vi "TCP_open.vi"(9 "timeout ms":i32=10000 caption="超时毫秒", 11 "Port":u16=2011 caption="端口") -> (0 "error IO":errorcluster, 1 "remote port":u16 caption="远程端口", 2 "remote address":string caption="远程地址", 3 "connection ID":refnum<k5>)   [LabVIEW 2013]
panel:
  # "通信接中～～～"
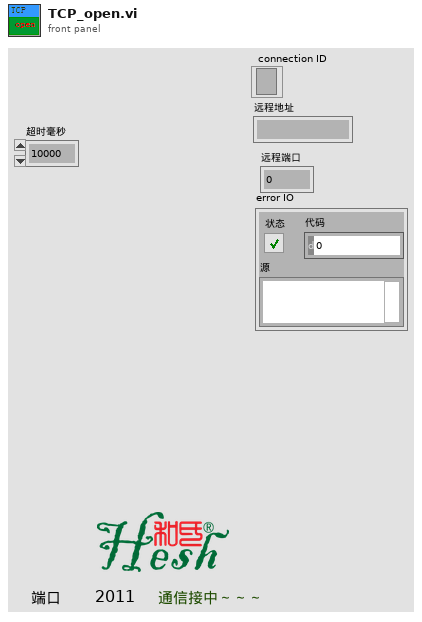
[diagram p1: front panel]
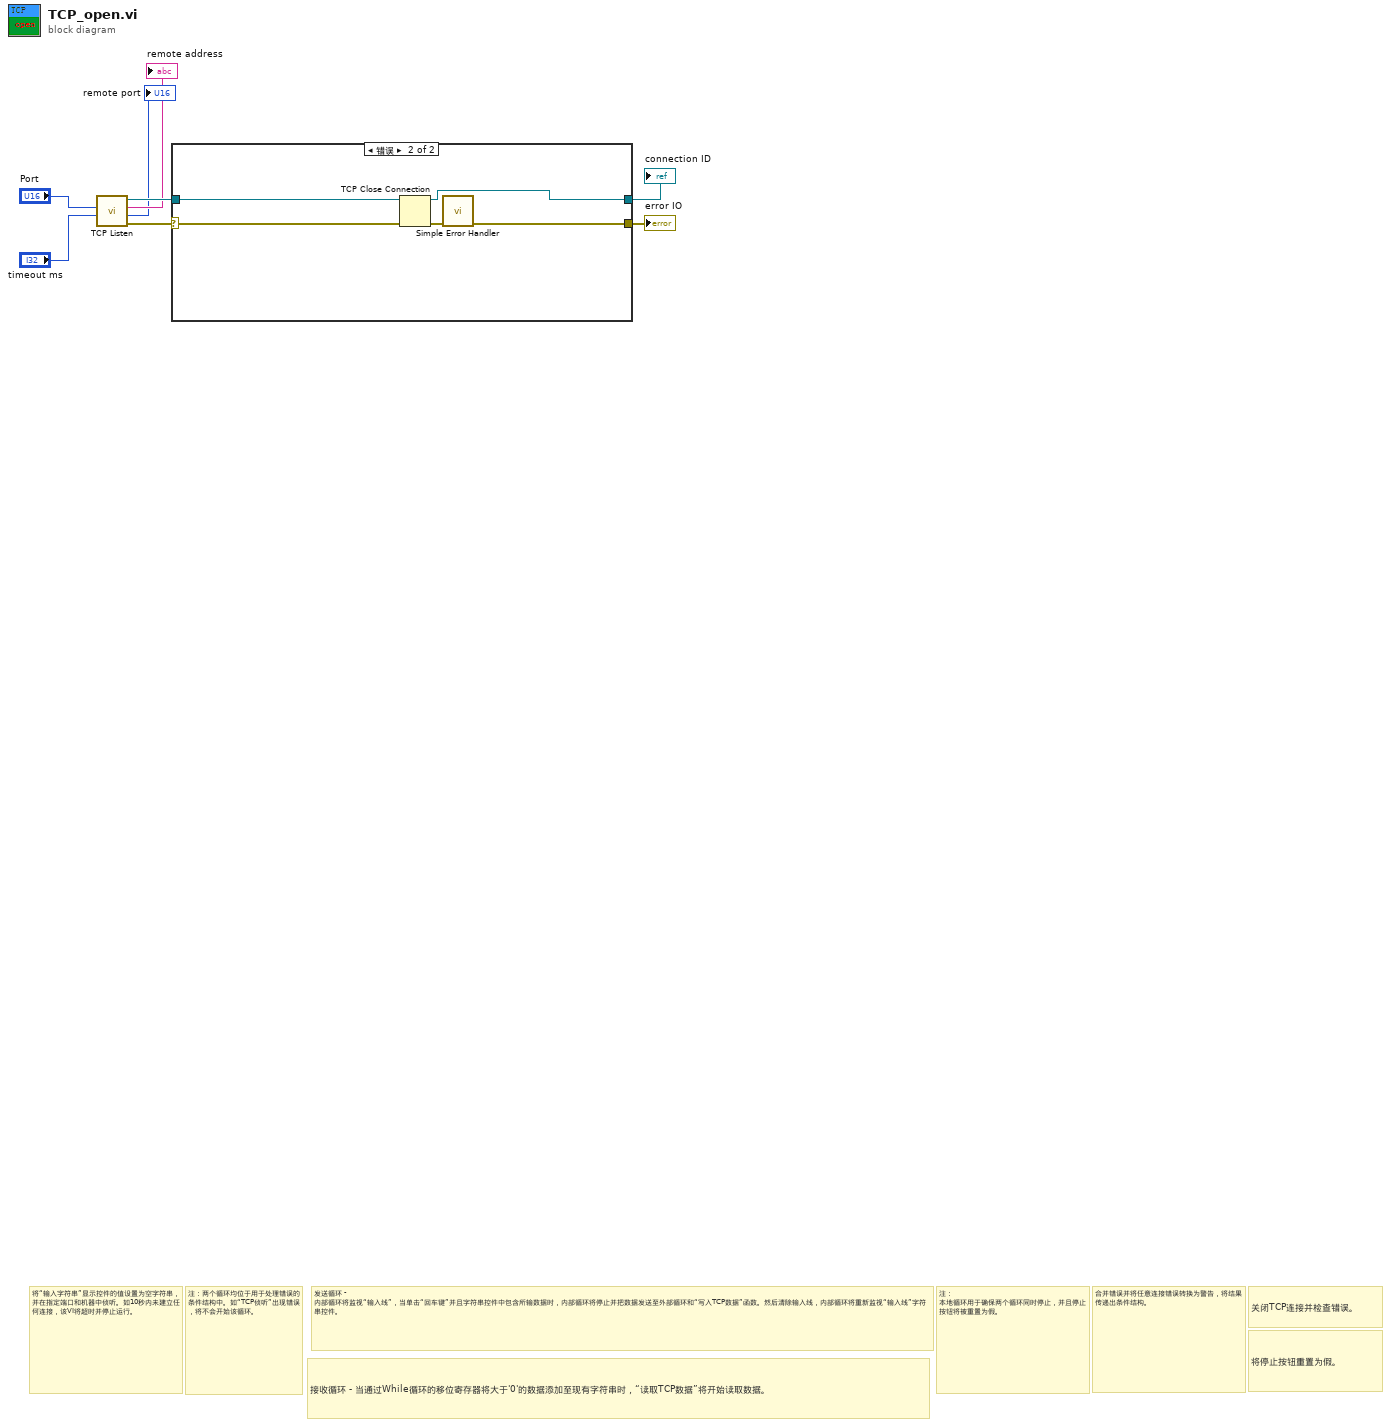
[diagram p0: block diagram]
diagram:
  # "将停止按钮重置为假。"
  # "关闭TCP连接并检查错误。"
  # "注：两个循环均位于用于处理错误的条件结构中。如“TCP侦听”出现错误，将不会开始该循环。"
  # "合并错误并将任意连接错误转换为警告，将结果传递出条件结构。"
  # "注： 本地循环用于确保两个循环同时停止，并且停止按钮将被重置为假。"
  # "接收循环 - 当通过While循环的移位寄存器将大于'0'的数据添加至现有字符串时，“读取TCP数据”将开始读取数据。"
  # "发送循环 - 内部循环将监视“输入线”，当单击“回车键”并且字符串控件中包含所输数据时，内部循环将停止并把数据发送至外部循环和“写入TCP数据”函数。然后清除输入线，内部循环将重新监视“输入线”字符串控件。"
  # "将“输入字符串”显示控件的值设置为空字符串，并在指定端口和机器中侦听。如10秒内未建立任何连接，该VI将超时并停止运行。"
  n1 = call <vilib>:"TCP Listen.vi"("timeout ms (wait forever: -1)"="timeout ms", "port"="Port") -> ("error out"=w7:errorcluster, "remote port"=→"remote port":u16, "remote address"=→"remote address":string, "connection ID"=w8:refnum<k5>)  [unwired: 5 in, 1 out]
  n2 = case shown="错误" w7 {
    selector: w7 -> [w10 w14]
    tunnel: w8 -> [w9 w13]
    tunnel: [w10 w12] -> w5
    tunnel: [w9 w11] -> w4
    frame No Error {
    }
    frame Error {
      n3 = TCP Close Connection(connection ID=w13, error in (no error)=w14) -> (connection ID out=w11:refnum<k5>, error out=w15:errorcluster)  [unwired: 1 in]
      n4 = call <vilib>:"Simple Error Handler.vi"("error in (no error)"=w15) -> ("error out"=w12:errorcluster)  [unwired: 4 in, 4 out]
    }
  }
  "error IO" <- w5
  "connection ID" <- w4
